vi "setModel.vi"(10 "Model":refnum<class "Model.lvclass">, 11 "Context in":refnum<class "Context.lvclass">) -> (3 "Context out":refnum<class "Context.lvclass">)   [LabVIEW 2016, in "Context.lvclass"]
uses:
  Context.lvclass
  Model/Model.lvclass
  Context.lvclass/Context.ctl
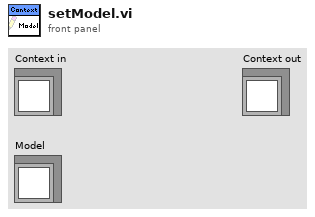
[diagram p1: front panel]
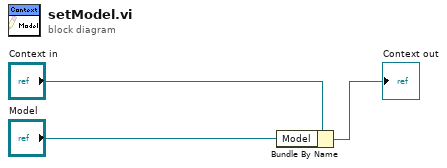
[diagram p0: block diagram]
diagram:
  n1 = Bundle By Name(cluster="Context in", "Model"="Model") -> (→"Context out":refnum<class "Context.lvclass">)
